vi "Alaram Histroy.vi"(7 "error IO":errorcluster, 8 "CodeMessage":string, 10 "Category":string(combo)="File Error", 11 "Tbl引用句柄":refnum<vi>) -> ()   [LabVIEW 2017]
panel:
  in  "Alaram History":string[][](table)=[["11F4", "0001", "D500"], ["11F6", "0001", "D502"], ["11F8", "0001", "D504"], ["11FC", "0001", "D508"], ["11FE", "0001", "D510"], ["1208", "0001", "D520"], ["0864", "0001", "M100"], ["0865", "0001", "M101"], ["0866", "0001", "M102"], ["0867", "0001", "M103"], ["0868", "0001", "M104"], ["0869", "0001", "M105"], ["086A", "0001", "M106"], ["086B", "0001", "M107"], ["086C", "0001", "M108"], ["1064", "0001", "D100"], ["1066", "0001", "D102"], ["1068", "0001", "D104"], ["106A", "0001", "D106"], ["0832", "0001", "M50"], ["0833", "0001", "M51"], ["0834", "0001", "M52"], ["0835", "0001", "M53"], ["0836", "0001", "M54"]]
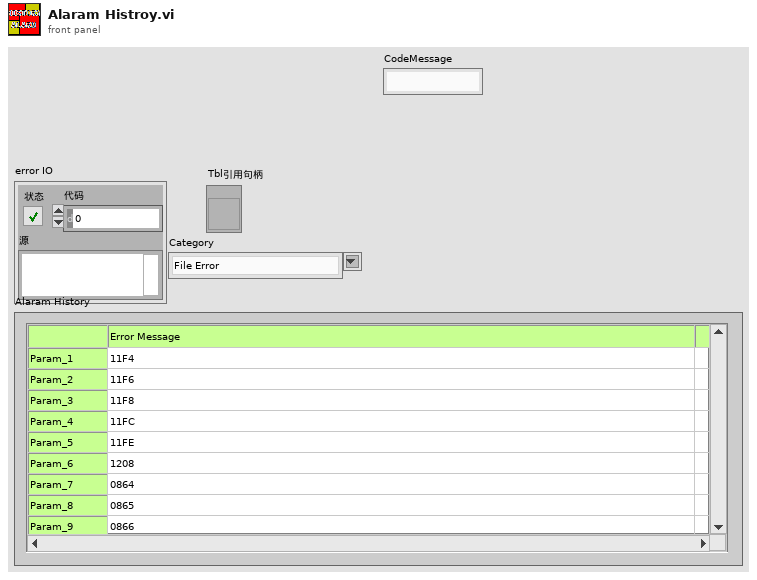
[diagram p1: front panel]
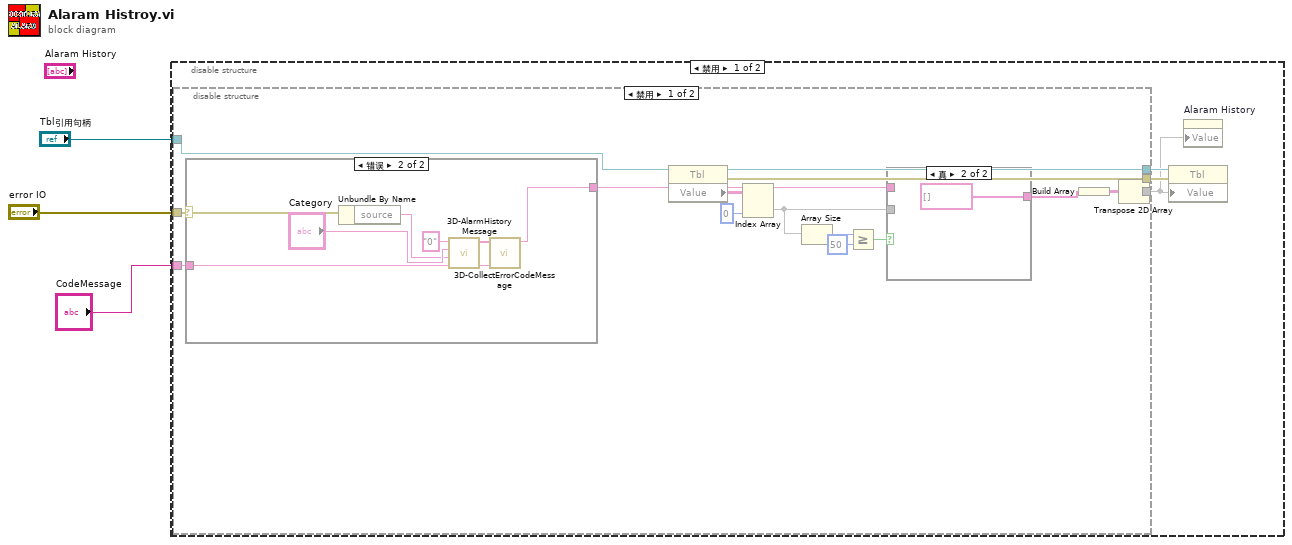
[diagram p0: block diagram]
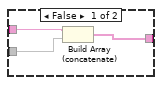
[diagram p2: hidden frame]
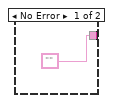
[diagram p3: hidden frame]
diagram:
  n1 = disable-structure shown="禁用" {
    disable-tunnel: "error IO" -> [w9 _]
    disable-tunnel: "Tbl引用句柄" -> [w8 _]
    disable-tunnel: "CodeMessage" -> [w4 _]
    frame Disabled {
      n2 = disable-structure shown="禁用" {
        disable-tunnel: w9 -> [w24 _]
        disable-tunnel: w8 -> [w23 _]
        disable-tunnel: [w20 _] -> w7
        disable-tunnel: [w19 _] -> w6
        disable-tunnel: [w17 _] -> w5
        disable-tunnel: w4 -> [w12 _]
        frame Disabled {
          n3 = case shown="错误" w24 {
            selector: w24 -> [_ w34]
            tunnel: ["" w32] -> w10
            tunnel: w12 -> [_ w30]
            frame No Error {
            }
            frame Error {
              n4 = Unbundle By Name(w34) -> ("source"=w33:string)
              n5 = call "3D-AlarmHistoryMessage.vi"("Duration"=w33, "Category"="Category", "Code"="0") -> ("AlarmMessage"=w31:string[])  [unwired: 8 in]
              n6 = call "3D-CollectErrorCodeMessage.vi"("Codemessage"=w30, "ErrorMessage"=w31) -> ("Error Code Message"=w32:string)  [unwired: 9 in]
            }
          }
          n7 = property class="Tbl"(reference=w23) -> (reference out=w20:refnum<vi>, error out=w19:errorcluster, "Value"=w22:string[][])  [unwired: 1 in]
          n8 = Index Array(array=w22, index (col)=0 ("禁用的索引 (列)")) -> (element=w13:string[])  [unwired: 1 in]
          n9 = Array Size(array=w13) -> (size(s)=w16:i32)
          n10 = Greater Or Equal?(x=w16, y=50) -> (x >= y?=w14:bool)
          n11 = case shown="真" w14 {
            tunnel: w13 -> [w26 _]
            tunnel: [w25 string[] [] ("Value")] -> w11
            tunnel: w10 -> [w27 _]
            frame False {
              n12 = Build Array (concatenate)(w27, w26) -> (w25:string[])
            }
            frame True {
            }
          }
          n13 = Build Array(w11) -> (w18:string[][])
          n14 = Transpose 2D Array(2D array=w18) -> (transposed array=w17:string[][])
        }
        frame Enabled {
        }
      }
      n15 = property class="Tbl"(reference=w7, error in=w6, "Value"=w5) -> ()  [unwired: 2 out]
      n16 = property on="Alaram History" class="Tbl (严格)"("Value"=w5) -> ()  [unwired: 2 in, 2 out]
    }
    frame Enabled {
    }
  }
